vi "save_metadata.vi"(8 "Cluster de Dados de Entrada":T1={"Corrente Inicial (mA)"=30.0, "Limite de Temperatura"=27.0, "Temperatura"=25.0, "Corrente Limite (mA)"=300, "Centralizar pico (nm)"=1557.0, "Valor de Span (nm)"=20.0, "Passo (mA)"=10.0, "Corrente Final (mA)"=650.0, "Resolucao"=enum."High"} {"Corrente Final (mA)" min=0.0 step=1.0; "Passo (mA)" min=1.0 step=1.0; "Valor de Span (nm)" min=0.1 max=1400.0 format="%.2f"; "Centralizar pico (nm)" format="%.2f"; "Temperatura" min=-100.0 max=199.9 step=0.1; "Limite de Temperatura" min=-100.0 max=199.9 step=0.1; "Corrente Inicial (mA)" min=0.0 step=1.0}, 11 "Pasta Destino":path=path "d:/Users/Stinky/Documents/11.04.2019/aquisicao14_HR_4mA_151_500") -> ()   [LabVIEW 2018]
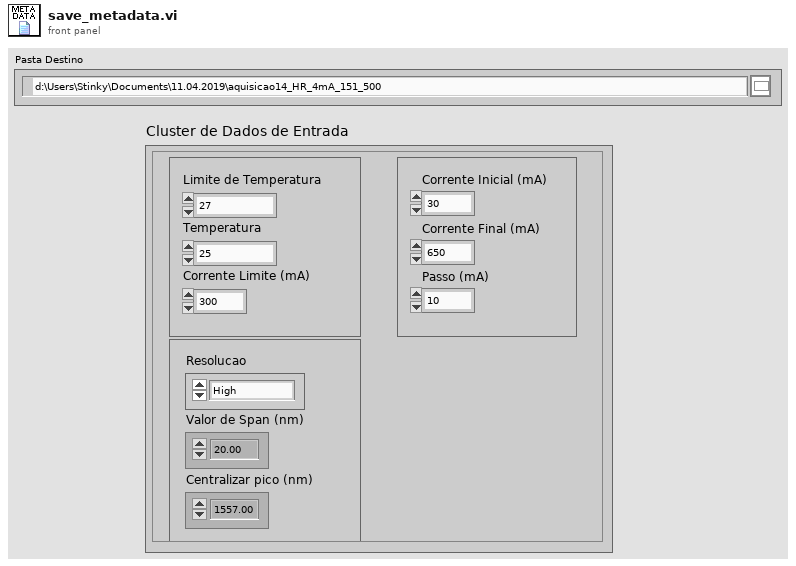
[diagram p1: front panel]
types:
  T1 = cluster{"Corrente Inicial (mA)":dbl, "Limite de Temperatura":dbl, "Temperatura":dbl, "Corrente Limite (mA)":i32, "Centralizar pico (nm)":dbl, "Valor de Span (nm)":dbl, "Passo (mA)":dbl, "Corrente Final (mA)":dbl, "Resolucao":enum16{"Normal", "High"}}
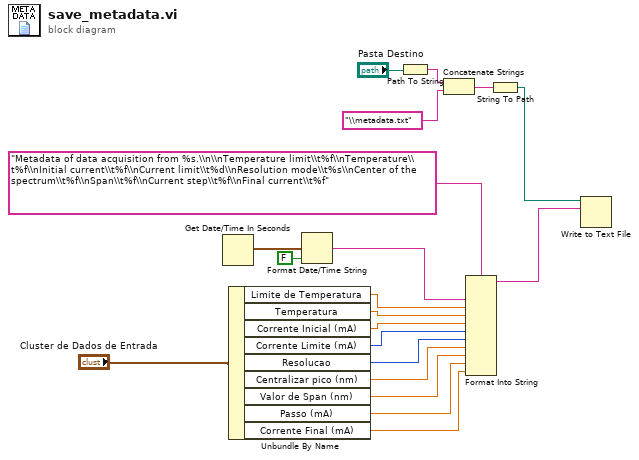
[diagram p0: block diagram]
diagram:
  n1 = Get Date/Time In Seconds() -> (seconds since 1Jan1904=w19:timestamp)
  n2 = Unbundle By Name("Cluster de Dados de Entrada") -> ("Limite de Temperatura"=w17:dbl, "Temperatura"=w16:dbl, "Corrente Inicial (mA)"=w15:dbl, "Corrente Limite (mA)"=w14:i32, "Resolucao"=w13:enum16{"Normal", "High"}, "Centralizar pico (nm)"=w12:dbl, "Valor de Span (nm)"=w11:dbl, "Passo (mA)"=w10:dbl, "Corrente Final (mA)"=w9:dbl)
  n3 = Format Date/Time String(seconds (now)=w19, UTC format=FALSE) -> (date/time string=w18:string)  [unwired: 1 in]
  n4 = Path To String(path="Pasta Destino") -> (string=w5:string)
  n5 = Concatenate Strings(w5, "\\metadata.txt") -> (w3:string)
  n6 = Format Into String(format string="Metadata of data acquisition from %s.\\n\\nTemperature limit\\t%f\\nTemperature\\t%f\\nInitial current\\t%f\\nCurrent limit\\t%d\\nResolution mode\\t%s\\nCenter of the spectrum\\t%f\\nSpan\\t%f\\nCurrent step\\t%f\\nFinal current\\t%f", w18, w17, w16, w15, w14, w13, w12, w11, w10, w9) -> (resulting string=w20:string)  [unwired: 2 in, 1 out]
  n7 = String To Path(string=w3) -> (path=w2:path)
  n8 = Write to Text File(file (use dialog)=w2, text=w20) -> ()  [unwired: 2 in, 3 out]
